vi "ArmGetCargoLoopPosition.vi"(1 "ArmAbsolutePose":T1, 2 "RobotDimensions":T2) -> (0 "CargoLoopPoints":cluster{dbl[], dbl[]})   [LabVIEW 2018]
uses:
  TypeDefs/ConfigComponents/Config_Dimensions.ctl
  TypeDefs/ArmAbsolutePosition.ctl
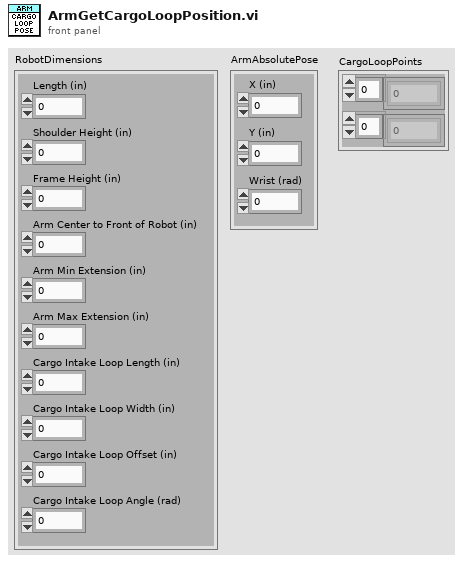
[diagram p1: front panel]
types:
  T1 = typedef "ArmAbsolutePosition.ctl" = cluster{"X (in)":dbl, "Y (in)":dbl, "Wrist (rad)":dbl}
  T2 = typedef "Config_Dimensions.ctl" = cluster{"Length (in)":dbl, "Shoulder Height (in)":dbl, "Frame Height (in)":dbl, "Arm Center to Front of Robot (in)":dbl, "Arm Min Extension (in)":dbl, "Arm Max Extension (in)":dbl, "Cargo Intake Loop Length (in)":dbl, "Cargo Intake Loop Width (in)":dbl, "Cargo Intake Loop Offset (in)":dbl, "Cargo Intake Loop Angle (rad)":dbl}
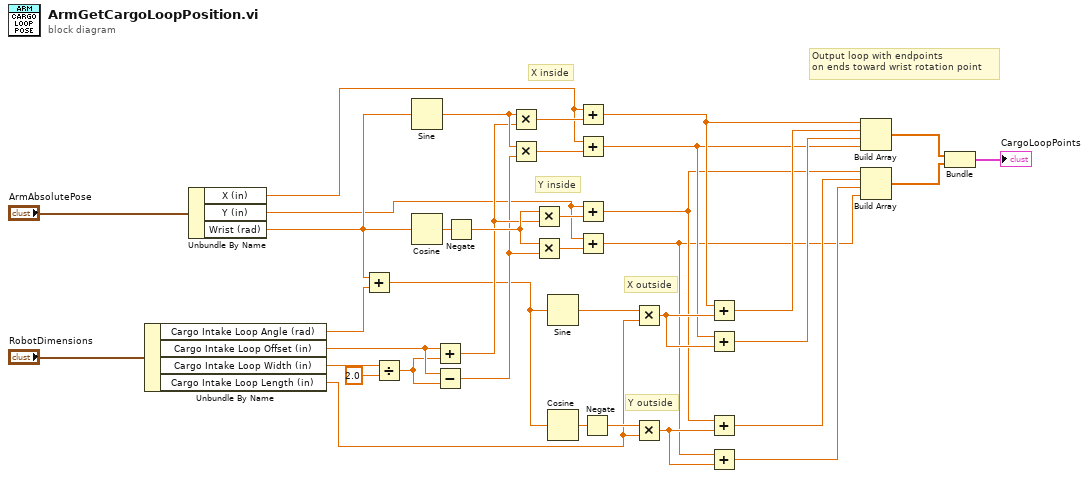
[diagram p0: block diagram]
diagram:
  # "Output loop with endpoints\non ends toward wrist rotation point"
  # "Y outside"
  # "X outside"
  # "Y inside"
  # "X inside"
  n1 = Unbundle By Name("RobotDimensions") -> ("Cargo Intake Loop Angle (rad)"=w35:dbl, "Cargo Intake Loop Offset (in)"=w32:dbl, "Cargo Intake Loop Width (in)"=w34:dbl, "Cargo Intake Loop Length (in)"=w14:dbl)
  n2 = Unbundle By Name("ArmAbsolutePose") -> ("X (in)"=w26:dbl, "Y (in)"=w19:dbl, "Wrist (rad)"=w29:dbl)
  n3 = Add(x=w29, y=w35) -> (x+y=w17:dbl)
  n4 = Divide(x=w34, y=2.0) -> (x/y=w31:dbl)
  n5 = Sine(x=w29) -> (sin(x)=w28:dbl)
  n6 = Cosine(x=w29) -> (cos(x)=w30:dbl)
  n7 = Add(x=w32, y=w31) -> (x+y=w21:dbl)
  n8 = Subtract(x=w32, y=w31) -> (x-y=w20:dbl)
  n9 = Negate(x=w30) -> (-x=w22:dbl)
  n10 = Multiply(x=w28, y=w21) -> (x*y=w27:dbl)
  n11 = Multiply(x=w28, y=w20) -> (x*y=w25:dbl)
  n12 = Multiply(x=w22, y=w21) -> (x*y=w23:dbl)
  n13 = Multiply(x=w22, y=w20) -> (x*y=w24:dbl)
  n14 = Sine(x=w17) -> (sin(x)=w16:dbl)
  n15 = Cosine(x=w17) -> (cos(x)=w18:dbl)
  n16 = Add(x=w26, y=w27) -> (x+y=w11:dbl)
  n17 = Add(x=w26, y=w25) -> (x+y=w8:dbl)
  n18 = Add(x=w19, y=w23) -> (x+y=w7:dbl)
  n19 = Add(x=w19, y=w24) -> (x+y=w4:dbl)
  n20 = Negate(x=w18) -> (-x=w15:dbl)
  n21 = Multiply(x=w16, y=w14) -> (x*y=w12:dbl)
  n22 = Multiply(x=w15, y=w14) -> (x*y=w13:dbl)
  n23 = Add(x=w11, y=w12) -> (x+y=w10:dbl)
  n24 = Add(x=w8, y=w12) -> (x+y=w9:dbl)
  n25 = Add(x=w7, y=w13) -> (x+y=w6:dbl)
  n26 = Add(x=w4, y=w13) -> (x+y=w5:dbl)
  n27 = Build Array(w11, w10, w9, w8) -> (w3:dbl[])
  n28 = Build Array(w7, w6, w5, w4) -> (w2:dbl[])
  n29 = Bundle(w3, w2) -> (→"CargoLoopPoints":cluster{dbl[], dbl[]})  [unwired: 1 in]
